vi "LaserTest.vi"() -> ()   [LabVIEW 2016, in "Laser Diode Controller.lvlib" / "KLD101.lvclass"]
uses:
  KLD101.lvclass
  Collimation/Components/Config Data/TypeDefs/LaserSettings.ctl
  Collimation/Components/Config Data/TypeDefs/LaserMode.ctl
  Collimation/Components/Config Data/TypeDefs/LaserPolarity.ctl
  Collimation/Components/Config Data/TypeDefs/LaserRampMode.ctl
  Collimation/Components/Config Data/Config Data.lvclass
panel:
  out "error out":errorcluster
  in  "dllPath":path=path "C:/Data/SVN/Projects/IDEXX/ProCyte Laser Fixture Software/Software/shared/ThorLabs/KLD101/Dependencies/Thorlabs.MotionControl.KCube.LaserDiode.dll"
  in  "stop":bool
  in  "laserOn":bool
  out "powerReading":dbl
  in  "serialNumber":string="98102964"
  in  "laserSettings":T1={"mode"=enum."Constant Current", "polarity"=enum."Cathode Grounded", "maxCurrent"=100, "pdFactor"=1.0, "rampMode"=enum."Immediate", "controlSrc"=enum."Software Only", "diodePower"=10.0, "swPowerScaling"=0.0, "diodeCurrent"=50.0}
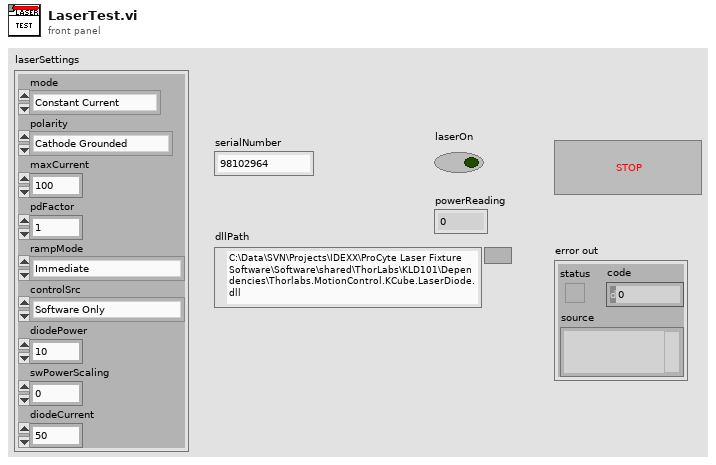
[diagram p1: front panel]
types:
  T1 = typedef "Configuration.lvlib/Config Data.lvclass/LaserSettings.ctl" = cluster{"mode":T2, "polarity":T3, "maxCurrent":i16, "pdFactor":sgl, "rampMode":T4, "controlSrc":enum16{"Software Only", "External Signal", "Potentiometer"}, "diodePower":dbl, "swPowerScaling":dbl, "diodeCurrent":dbl}
  T2 = typedef "Configuration.lvlib/Config Data.lvclass/LaserMode.ctl" = enum16{"Constant Power", "Constant Current"}
  T3 = typedef "Configuration.lvlib/Config Data.lvclass/LaserPolarity.ctl" = enum16{"Anode Grounded", "Cathode Grounded"}
  T4 = typedef "Configuration.lvlib/Config Data.lvclass/LaserRampMode.ctl" = enum16{"Immediate", "Ramped"}
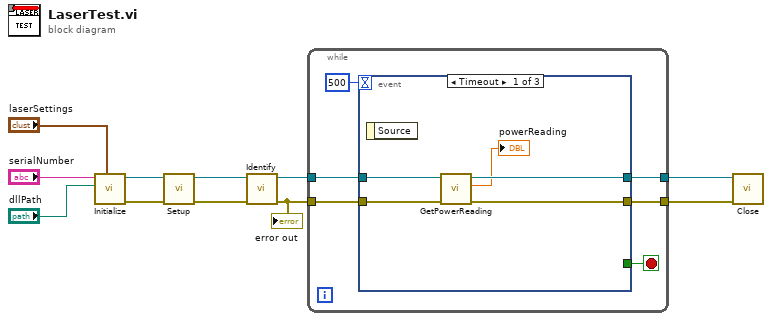
[diagram p0: block diagram]
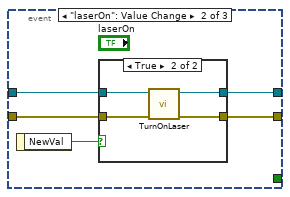
[diagram p2: hidden frame]
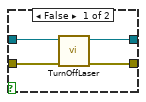
[diagram p3: hidden frame]
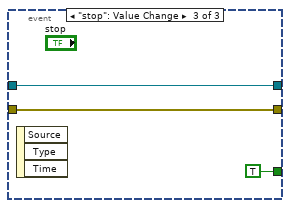
[diagram p4: hidden frame]
diagram:
  n1 = call "Initialize.vi"("laserSettings"="laserSettings", "dllPath"="dllPath", "serialNumber"="serialNumber") -> ("error out"=w9:errorcluster, "Laser Diode Controller out"=w10:refnum<class "KLD101.lvclass">)  [unwired: 7 in]
  n2 = call-dynamic "Setup.vi"("error in (no error)"=w9, "Laser Diode Controller in"=w10) -> ("error out"=w2:errorcluster, "Laser Diode Controller out"=w8:refnum<class "KLD101.lvclass">)  [unwired: 8 in]
  n3 = call-dynamic "Identify.vi"("error in (no error)"=w2, "Laser Diode Controller in"=w8) -> ("error out"=w5:errorcluster, "Laser Diode Controller out"=w6:refnum<class "KLD101.lvclass">)  [unwired: 8 in]
  "error out" <- w5
  n4 = while {
    tunnel: [w17] -> w4
    tunnel: w6 -> [w16]
    tunnel: [w15] -> w3
    tunnel: w5 -> [w14]
    stop <- w12 stop-if-true
    n5 = event shown="[0] Timeout" {
      selector: _ -> [_ _ _]
      dyn-events: _ -> [_ _ _]
      timeout: 500 -> [_ _ _]
      tunnel: [w21 w25 w38] -> w17
      tunnel: w16 -> [w22 w26 w38]
      tunnel: [w19 w23 w37] -> w15
      tunnel: w14 -> [w20 w24 w37]
      tunnel: [_ _ TRUE] -> w12
      event Timeout {
        n6 = event-data() -> ()  [unwired: 1 in, 1 out]
        n7 = call-dynamic "GetPowerReading.vi"("error in (no error)"=w20, "Laser Diode Controller in"=w22) -> ("error out"=w19:errorcluster, "powerReading"=→"powerReading":dbl, "Laser Diode Controller out"=w21:refnum<class "KLD101.lvclass">)  [unwired: 7 in]
      }
      event "laserOn": Value Change {
        n8 = event-data() -> ("NewVal"=w27:bool)  [unwired: 1 in]
        n9 = case shown="True" w27 {
          tunnel: w26 -> [w31 w35]
          tunnel: [w30 w34] -> w25
          tunnel: w24 -> [w29 w33]
          tunnel: [w28 w32] -> w23
          frame False {
            n10 = call-dynamic "TurnOffLaser.vi"("error in (no error)"=w29, "Laser Diode Controller in"=w31) -> ("error out"=w28:errorcluster, "Laser Diode Controller out"=w30:refnum<class "KLD101.lvclass">)  [unwired: 8 in]
          }
          frame True {
            n11 = call-dynamic "TurnOnLaser.vi"("error in (no error)"=w33, "Laser Diode Controller in"=w35) -> ("error out"=w32:errorcluster, "Laser Diode Controller out"=w34:refnum<class "KLD101.lvclass">)  [unwired: 8 in]
          }
        }
      }
      event "stop": Value Change {
        n12 = event-data() -> ()  [unwired: 1 in, 3 out]
      }
    }
  }
  n13 = call-dynamic "Close.vi"("error in (no error)"=w3, "Laser Diode Controller in"=w4) -> ()  [unwired: 9 in, 1 out]
